vi "AngR.vi"() -> ()   [LabVIEW 2018]
uses:
  <vilib>/Utility/file.llb/Write Delimited Spreadsheet (DBL).vi
panel:
  out "Potenciometro":dbl[](graph)
  in  "test":bool
  in  "Nombre":string
  out "Ind":i32
  out "Angulo":dbl
  out "R 4":cluster{"Array":dbl[], dbl[]}(graph)
  out "R 1":cluster{dbl[], dbl[]}(graph)
  in  "Medir  R":bool
  in  "Medir  P":bool
  in  "Paso":dbl
  in  "Ang End":dbl
  in  "Ang inicio":dbl
  in  "stop":bool
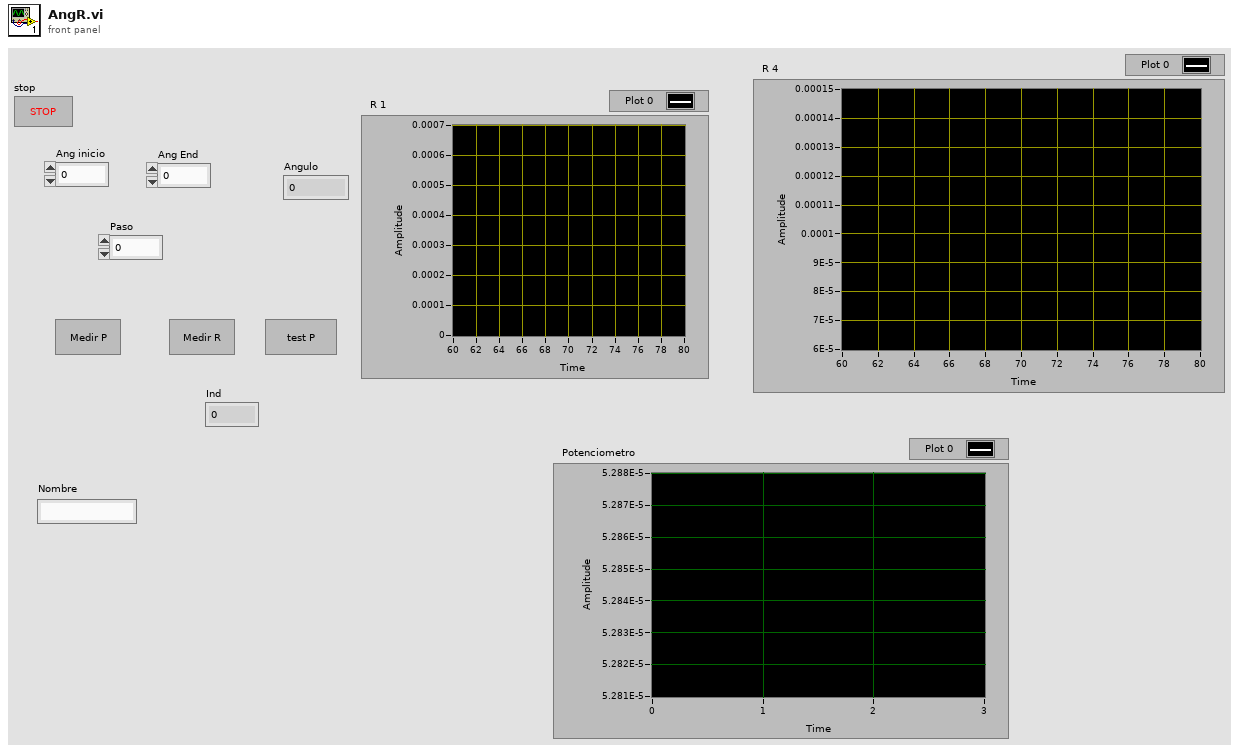
[diagram p1: front panel]
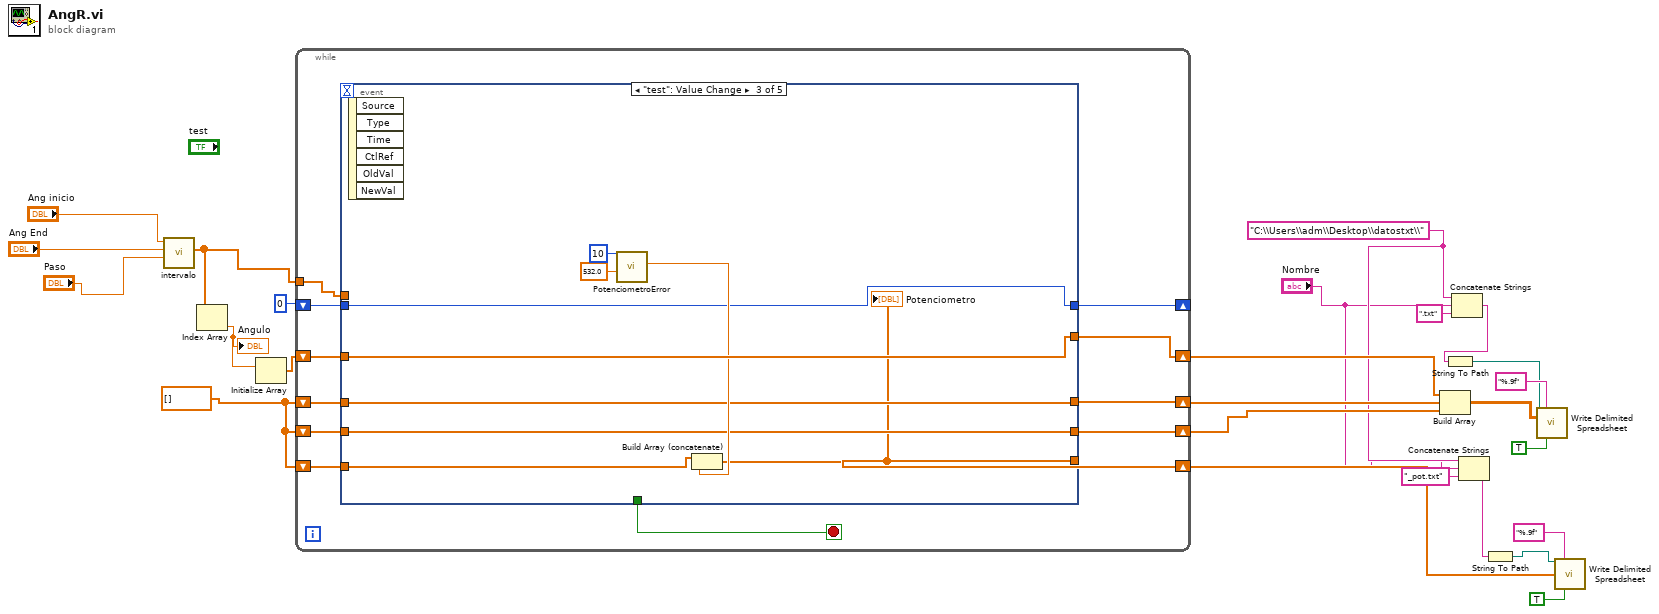
[diagram p0: block diagram]
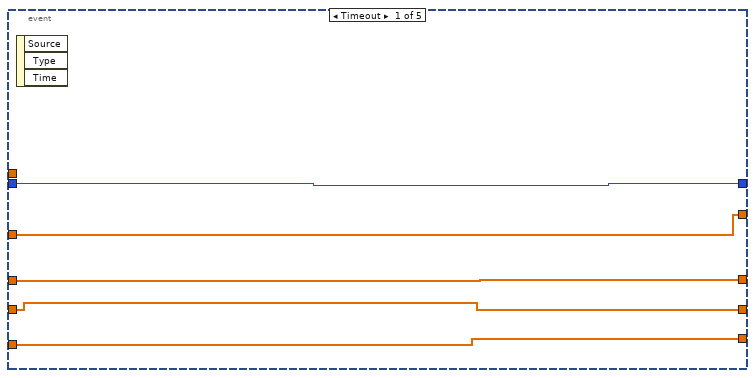
[diagram p2: hidden frame]
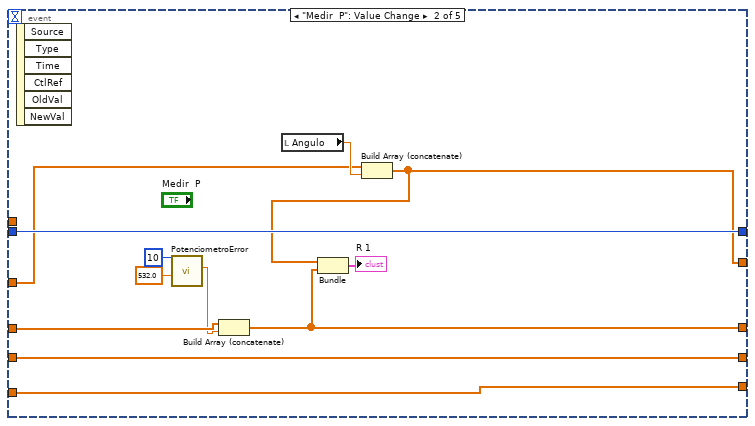
[diagram p3: hidden frame]
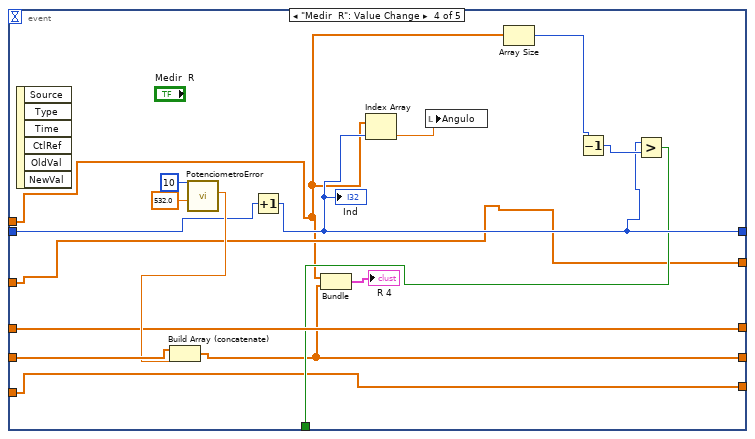
[diagram p4: hidden frame]
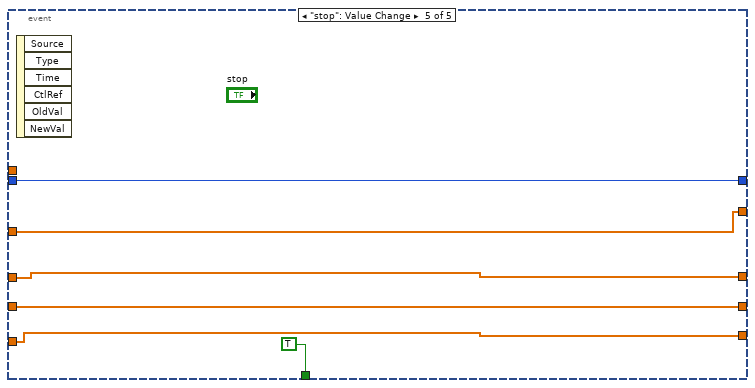
[diagram p5: hidden frame]
diagram:
  w5 = "C:\\Users\\adm\\Desktop\\datostxt\\"
  w22 = dbl[] []
  n1 = call "intervalo.vi"("incremento"="Paso", "fin"="Ang End", "inicio"="Ang inicio") -> ("Array"=w21:dbl[])  [unwired: 8 in]
  n2 = Index Array(array=w21) -> (element=w10:dbl)  [unwired: 1 in]
  "Angulo" <- w10
  n3 = Initialize Array(w10) -> (w11:dbl[])  [unwired: 1 in]
  n4 = while {
    tunnel: w21 -> [w30]
    shift-right: [w36] -> w19
    shift-left: w22 -> [w37]
    shift-right: [w35] -> w18
    shift-left: w22 -> [w34]
    shift-right: [w33] -> w6
    shift-left: w22 -> [w32]
    shift-right: [w28] -> _
    shift-left: 0 -> [w29]
    shift-right: [w26] -> w9
    shift-left: w11 -> [w27]
    stop <- w31 stop-if-true
    n5 = event shown="[2] \"test\": Value Change" {
      selector: _ -> [_ _ _ _ _]
      dyn-events: _ -> [_ _ _ _ _]
      timeout: _ -> [_ _ _ _ _]
      tunnel: w37 -> [w42 w54 w57 w75 w84]
      tunnel: [w42 w44 w57 w75 w84] -> w36
      tunnel: [w41 w50 w58 w65 w83] -> w35
      tunnel: w34 -> [w41 w50 w58 w77 w83]
      tunnel: [w40 w49 w56 w64 w82] -> w33
      tunnel: w32 -> [w40 w49 w60 w64 w82]
      tunnel: [_ _ _ w70 TRUE] -> w31
      tunnel: w30 -> [_ _ _ w66 _]
      tunnel: w29 -> [w39 w48 w55 w74 w81]
      tunnel: [w39 w48 w55 w71 w81] -> w28
      tunnel: w27 -> [w38 w46 w63 w68 w80]
      tunnel: [w38 w45 w63 w68 w80] -> w26
      event Timeout {
        n6 = event-data() -> ()  [unwired: 1 in, 3 out]
      }
      event "Medir  P": Value Change {
        n7 = event-data() -> ()  [unwired: 1 in, 6 out]
        n8 = call "PotenciometroError.vi"("Wavelength (0.0)"=532.0, "num Lect"=10) -> ("Valor Prom"=w51:dbl)  [unwired: 8 in, 1 out]
        n9 = Build Array (concatenate)(w54, w51) -> (w44:dbl[])
        n10 = local read "Angulo"() -> (w47:dbl)
        n11 = Build Array (concatenate)(w46, w47) -> (w45:dbl[])
        n12 = Bundle(w45, w44) -> (→"R 1":cluster{dbl[], dbl[]})  [unwired: 1 in]
      }
      event "test": Value Change {
        n13 = event-data() -> ()  [unwired: 1 in, 6 out]
        n14 = call "PotenciometroError.vi"("Wavelength (0.0)"=532.0, "num Lect"=10) -> ("Valor Prom"=w59:dbl)  [unwired: 8 in, 1 out]
        n15 = Build Array (concatenate)(w60, w59) -> (w56:dbl[])
        "Potenciometro" <- w56
      }
      event "Medir  R": Value Change {
        n16 = event-data() -> ()  [unwired: 1 in, 6 out]
        n17 = call "PotenciometroError.vi"("Wavelength (0.0)"=532.0, "num Lect"=10) -> ("Valor Prom"=w76:dbl)  [unwired: 8 in, 1 out]
        n18 = Build Array (concatenate)(w77, w76) -> (w65:dbl[])
        n19 = Increment(x=w74) -> (x+1=w71:i32)
        "Ind" <- w71
        n20 = Bundle("Array"=w66, w65) -> (→"R 4":cluster{"Array":dbl[], dbl[]})  [unwired: 1 in]
        n21 = Index Array(array=w66, index=w71) -> (element=w69:dbl)
        n22 = local write "Angulo"(w69) -> ()
        n23 = Array Size(array=w66) -> (size(s)=w72:i32)
        n24 = Decrement(x=w72) -> (x-1=w73:i32)
        n25 = Greater?(x=w71, y=w73) -> (0:w70:bool)
      }
      event "stop": Value Change {
        n26 = event-data() -> ()  [unwired: 1 in, 6 out]
      }
    }
  }
  n27 = Build Array(w9, w19, w18) -> (w17:dbl[][])
  n28 = Concatenate Strings(w5, "Nombre", ".txt" ("string")) -> (w14:string)
  n29 = String To Path(string=w14) -> (path=w13:path)
  n30 = Concatenate Strings(w5, "Nombre", "_pot.txt" ("string")) -> (w1:string)
  n31 = String To Path(string=w1) -> (path=w2:path)
  n32 = call-poly <vilib>:"Write Delimited Spreadsheet.vi"("file path (dialog if empty)"=w13, "format (%.3f)"="%.9f", "2D data"=w17, "transpose? (no:F)"=TRUE) -> ()  [unwired: 10 in, 2 out]
  n33 = call-poly <vilib>:"Write Delimited Spreadsheet.vi"("file path (dialog if empty)"=w2, "format (%.3f)"="%.9f", "1D data"=w6, "transpose? (no:F)"=TRUE) -> ()  [unwired: 10 in, 2 out]
